vi "Parse Excluded Tests on Items.vi"(8 "error in (no error)":errorcluster, 11 "ExcludedTestsOnItems Element":refnum<k20>) -> (0 "error out":errorcluster, 2 "Excluded Tests on Items":T1(array[cluster]))   [LabVIEW 2020]
uses:
  <vilib>/xml/Close Reference(Node).vi
  <vilib>/xml/NI_XML.lvlib
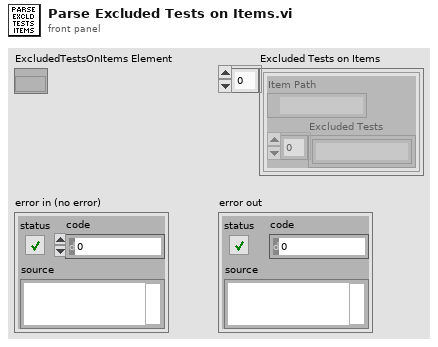
[diagram p1: front panel]
types:
  T1 = cluster{"Item Path":path, "Excluded Tests":string[]}[]
  T2 = cluster{"Item Path":path, "Excluded Tests":string[]}
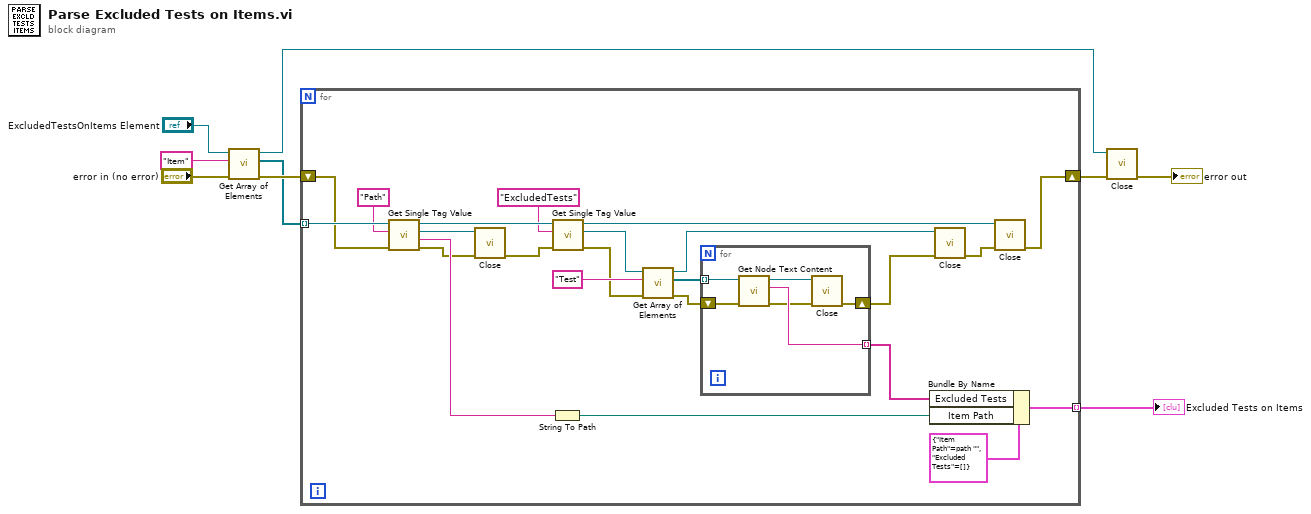
[diagram p0: block diagram]
diagram:
  n1 = call <vilib>:"Get Array of Elements.vi"("error in (no error)"="error in (no error)", "Tag Name"="Item", "Refnum in"="ExcludedTestsOnItems Element") -> ("error out"=w9:errorcluster, "Array Of Elements"=w8:refnum<k20>[], "Refnum out"=w7:refnum<k20>)  [unwired: 6 in]
  n2 = for {
    tunnel: w8 -> [w32] mode=indexing
    shift-right: [w27] -> w6
    shift-left: w9 -> [w31]
    tunnel: [w26] -> w1 mode=indexing
    n3 = call <vilib>:"Get Single Tag Value.vi"("Error In"=w31, "Tag Name"="Path", "Element In"=w32) -> ("Error Out"=w21:errorcluster, "Tag Value"=w23:string, "Tag Reference"=w22:refnum<k20>, "Element Out"=w30:refnum<k20>)  [unwired: 5 in]
    n4 = call-poly <vilib>:"Close.vi"("error in (no error)"=w21, "node"=w22) -> ("error out"=w19:errorcluster)  [unwired: 7 in]
    n5 = String To Path(string=w23) -> (path=w29:path)
    n6 = call <vilib>:"Get Single Tag Value.vi"("Error In"=w19, "Tag Name"="ExcludedTests", "Element In"=w30) -> ("Error Out"=w15:errorcluster, "Tag Reference"=w17:refnum<k20>, "Element Out"=w28:refnum<k20>)  [unwired: 5 in, 1 out]
    n7 = call <vilib>:"Get Array of Elements.vi"("error in (no error)"=w15, "Tag Name"="Test" ("Get Elements By Tag Name Array"), "Refnum in"=w17) -> ("error out"=w12:errorcluster, "Array Of Elements"=w14:refnum<k20>[], "Refnum out"=w10:refnum<k20>)  [unwired: 6 in]
    n8 = for {
      tunnel: w14 -> [w38] mode=indexing
      tunnel: [w36] -> w13 mode=indexing
      shift-right: [w33] -> w11
      shift-left: w12 -> [w35]
      n9 = call <vilib>:"Get Node Text Content.vi"("error in (no error)"=w35, "node in"=w38) -> ("error out"=w34:errorcluster, "node text"=w36:string, "node out"=w37:refnum<k20>)  [unwired: 7 in]
      n10 = call-poly <vilib>:"Close.vi"("error in (no error)"=w34, "node"=w37) -> ("error out"=w33:errorcluster)  [unwired: 7 in]
    }
    n11 = Bundle By Name(cluster=T2 {"Item Path"=path "", "Excluded Tests"=[]} ("Cluster"), "Excluded Tests"=w13, "Item Path"=w29) -> (w26:T2)
    n12 = call-poly <vilib>:"Close.vi"("error in (no error)"=w11, "node"=w10) -> ("error out"=w20:errorcluster)  [unwired: 7 in]
    n13 = call-poly <vilib>:"Close.vi"("error in (no error)"=w20, "node"=w28) -> ("error out"=w27:errorcluster)  [unwired: 7 in]
  }
  "Excluded Tests on Items" <- w1
  n14 = call-poly <vilib>:"Close.vi"("error in (no error)"=w6, "node"=w7) -> ("error out"=→"error out":errorcluster)  [unwired: 7 in]
